vi "Stream Test.vi"() -> ()   [LabVIEW 2015]
uses:
  DAQ Engine VIs/PXI Globals.vi
panel:
  out "Graph":dbl[][](graph)
  out "Pause?":bool
  in  "Pause":bool
  in  "Gate":T1={"Active"=TRUE, "Delay (ms)"=20.0, "Width (ms)"=100.0, "Ramp (ms)"=5.0}
  out "Abort":bool
  in  "START":bool
  in  "RETURN":bool
  in  "STOP":bool
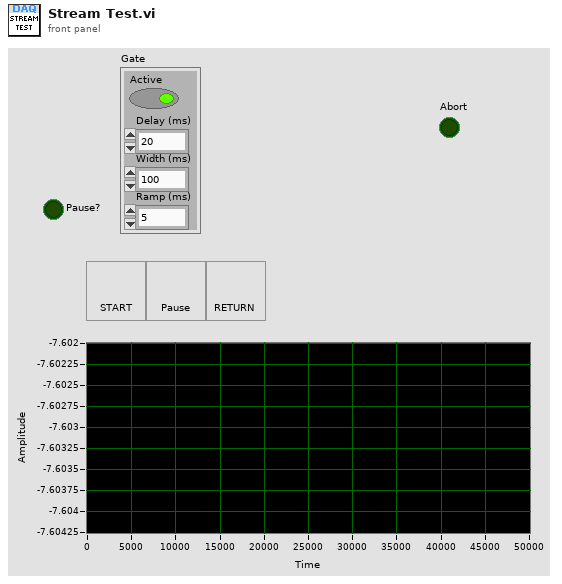
[diagram p1: front panel]
types:
  T1 = cluster{"Active":bool, "Delay (ms)":dbl, "Width (ms)":dbl, "Ramp (ms)":dbl}
  T2 = cluster{"Shift":bool, "Ctrl":bool, "Alt":bool, "Cmd":bool, "Opt":bool}
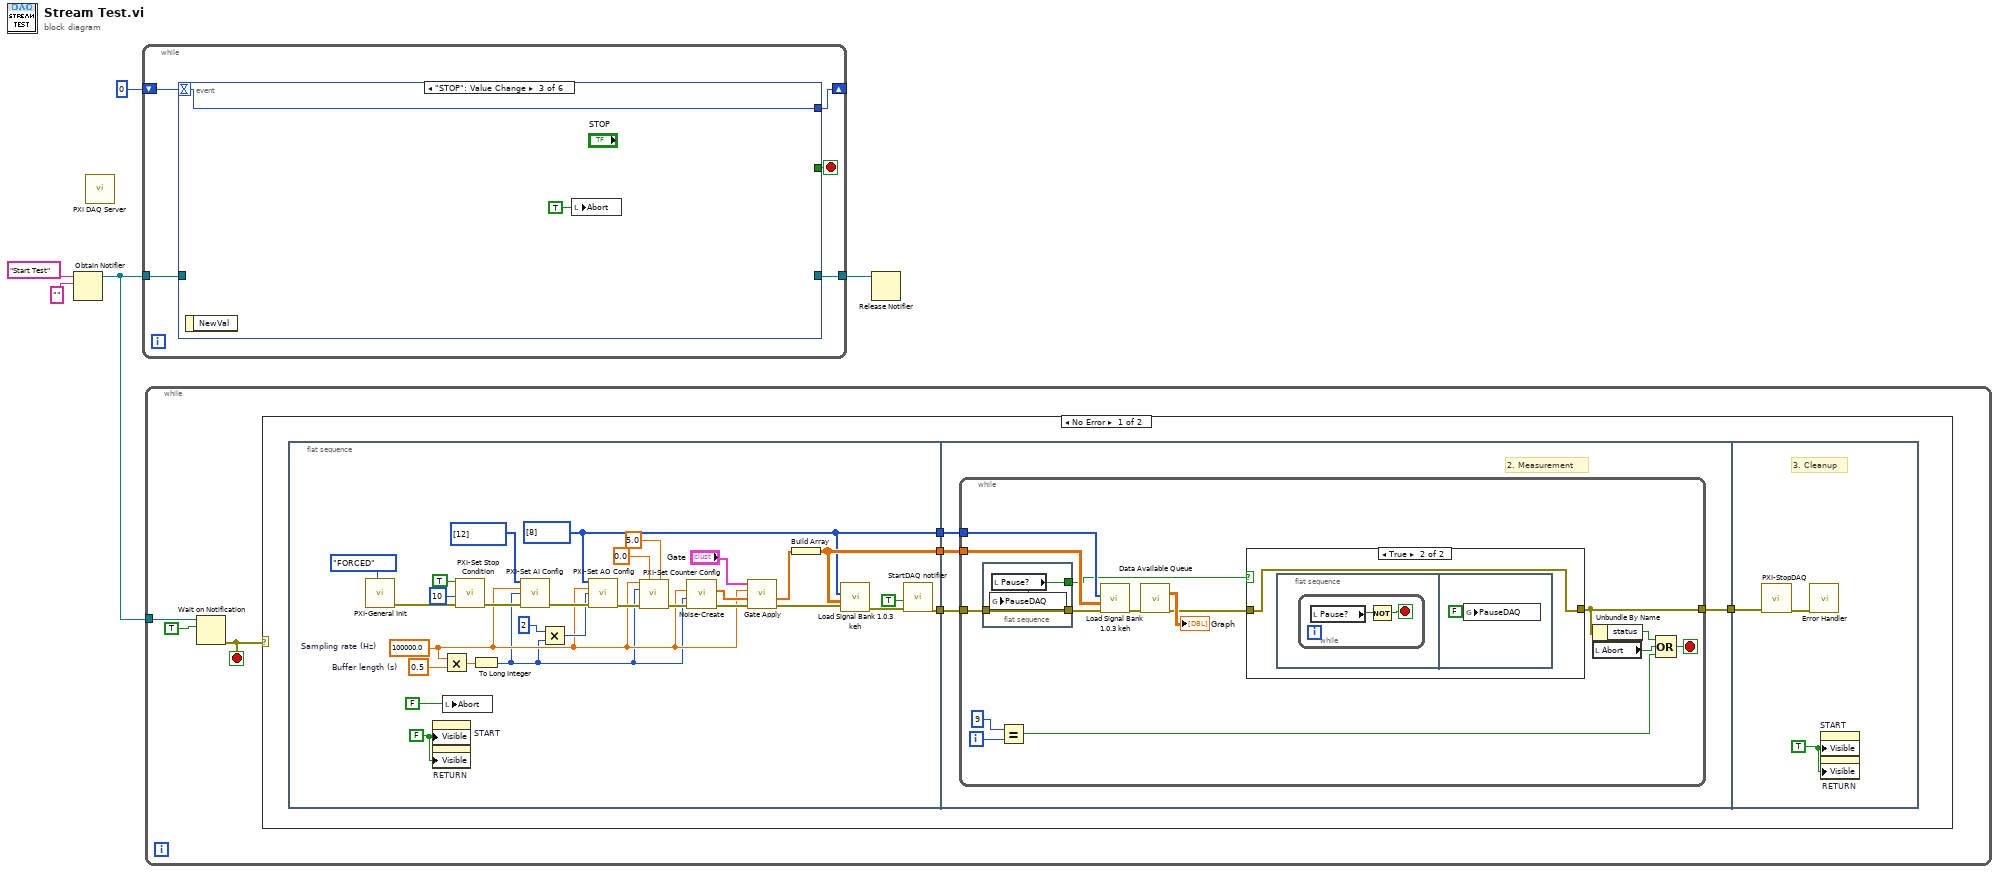
[diagram p0: block diagram]
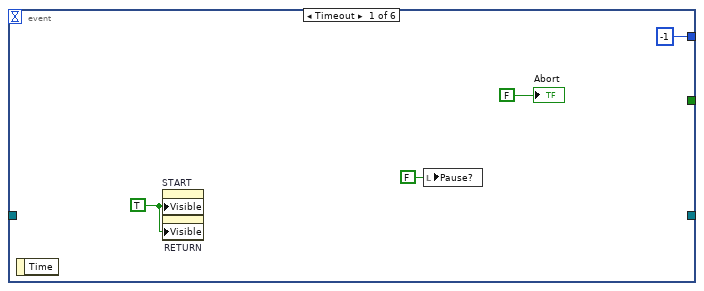
[diagram p4: hidden frame]
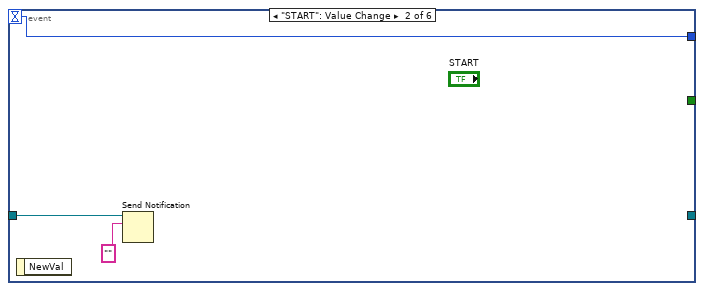
[diagram p5: hidden frame]
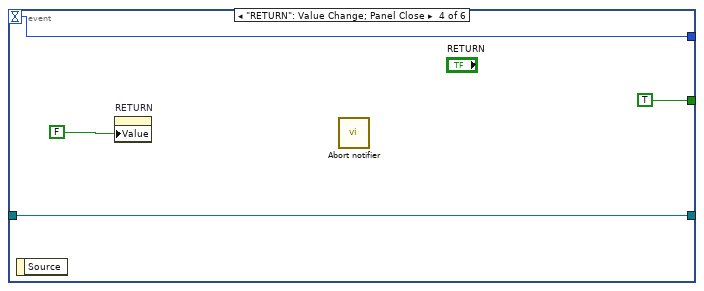
[diagram p6: hidden frame]
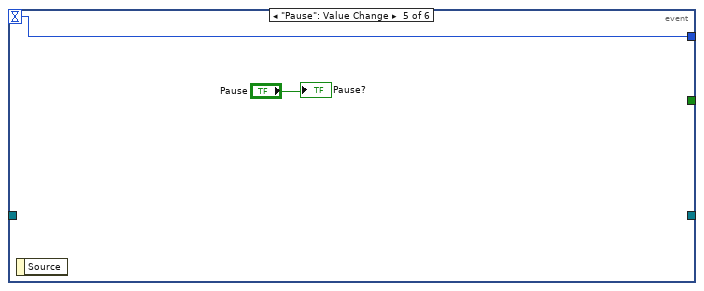
[diagram p7: hidden frame]
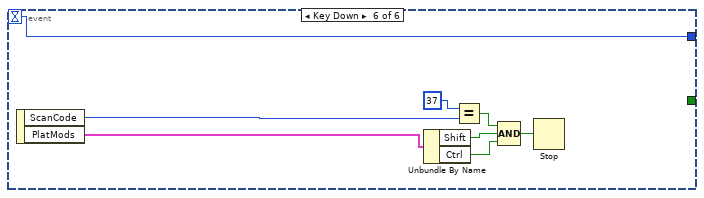
[diagram p8: hidden frame]
diagram:
  n1 = Obtain Notifier(name (unnamed)="Start Test", notification data type="") -> (notifier out=w5:refnum<notifier>)  [unwired: 2 in, 2 out]
  n2 = call "PXI DAQ Server.vi"() -> ()  [unwired: 7 in, 1 out]
  n3 = while {
    tunnel: w5 -> [w10]
    tunnel: [w8] -> w4
    shift-right: [w6] -> _
    shift-left: 0 -> [w7]
    stop <- w9 stop-if-true
    n4 = event shown="[2] \"STOP\": Value Change" {
      selector: _ -> [_ _ _ _ _ _]
      dyn-events: _ -> [_ _ _ _ _ _]
      timeout: w7 -> [_ w15 w18 w21 w25 w26]
      tunnel: w10 -> [_ w16 _ w22 _ _]
      tunnel: [_ _ _ TRUE _ _] -> w9
      tunnel: [_ _ _ w22 _ _] -> w8
      tunnel: [-1 w15 w18 w21 w25 w26] -> w6
      event Timeout {
        w12 = TRUE ("Visible")
        n5 = event-data() -> ()  [unwired: 1 in, 1 out]
        n6 = property on="START" class="Bool"("Visible"=w12) -> ()  [unwired: 2 in, 2 out]
        n7 = property on="RETURN" class="Bool (strict)"("Visible"=w12) -> ()  [unwired: 2 in, 2 out]
        n8 = local write "Pause?"(FALSE ("Pause?")) -> ()
        "Abort" <- FALSE ("Abort")
      }
      event "START": Value Change {
        n9 = event-data() -> ()  [unwired: 1 in, 1 out]
        n10 = Send Notification(notification="", notifier=w16) -> ()  [unwired: 1 in, 2 out]
      }
      event "STOP": Value Change {
        n11 = event-data() -> ()  [unwired: 1 in, 1 out]
        n12 = local write "Abort"(TRUE ("Global Abort")) -> ()
      }
      event "RETURN": Value Change; Panel Close {
        n13 = event-data() -> ()  [unwired: 1 in, 1 out]
        n14 = property on="RETURN" class="Bool (strict)"("Value"=FALSE) -> ()  [unwired: 2 in, 2 out]
        n15 = call "Abort notifier.vi"() -> ()  [unwired: 6 in, 2 out]
      }
      event "Pause": Value Change {
        n16 = event-data() -> ()  [unwired: 1 in, 1 out]
        "Pause?" <- "Pause"
      }
      event Key Down {
        n17 = event-data() -> ("ScanCode"=w28:i16, "PlatMods"=w27:T2)  [unwired: 1 in]
        n18 = Unbundle By Name(w27) -> ("Shift"=w31:bool, "Ctrl"=w30:bool)
        n19 = Equal?(x=i16 37 ("y"), y=w28) -> (x = y?=w32:bool)
        n20 = Compound Arithmetic op=AND(w32, w31, w30) -> (w29:bool)
        n21 = Stop(stop? (T)=w29) -> ()
      }
    }
  }
  n22 = while {
    tunnel: w5 -> [w35]
    stop <- w34 stop-if-true
    n23 = Wait on Notification(notifier=w35, ignore previous (F)=TRUE) -> (error out=w34:errorcluster)  [unwired: 2 in, 3 out]
    n24 = case shown="No Error" w34 {
      frame No Error {
        n25 = flat-sequence {
          tunnel: [w69] -> w40
          tunnel: [w49] -> w39
          tunnel: [w51] -> w38
          tunnel: w40 -> [w73]
          tunnel: w39 -> [w72]
          tunnel: w38 -> [w71]
          tunnel: [w70] -> w37
          tunnel: w37 -> [w96]
          frame #0 {
            w49 = i32[] [8] ("AI Channels")
            w58 = 0.5  # Buffer length (s)
            w44 = 100000.0  # Sampling rate (Hz)
            w68 = FALSE ("Visible")
            n26 = call "PXI-General Init.vi"("Double Buffer Mode"=enum32{"OFF", "ENABLED", "FORCED"}."FORCED") -> ("error out"=w59:errorcluster)  [unwired: 10 in]
            n27 = property on="START" class="Bool"("Visible"=w68) -> ()  [unwired: 2 in, 2 out]
            n28 = property on="RETURN" class="Bool (strict)"("Visible"=w68) -> ()  [unwired: 2 in, 2 out]
            n29 = Multiply(x=w44, y=w58) -> (x*y=w54:dbl)
            n30 = local write "Abort"(FALSE ("Global Abort")) -> ()
            n31 = call "PXI-Set Stop Condition.vi"("Stop on Max Presentations?"=TRUE, "Number of presentations"=10, "error in (no error)"=w59) -> ("error out"=w48:errorcluster)  [unwired: 12 in]
            n32 = To Long Integer(number=w54) -> (32bit integer=w43:i32)
            n33 = call "PXI-Set AI Config.vi"("AI Channels"=i32[] [12], "Sampling Rate (Hz)"=w44, "Buffer Size"=w43, "error in (no error)"=w48) -> ("error out"=w60:errorcluster)  [unwired: 11 in]
            n34 = Multiply(x=2, y=w43) -> (x*y=w56:i32)
            n35 = call "PXI-Set AO Config.vi"("AO Channels"=w49, "Sampling Rate (Hz)"=w44, "Buffer Size"=w56, "error in (no error)"=w60) -> ("error out"=w61:errorcluster)  [unwired: 11 in]
            n36 = call "PXI-Set Counter Config.vi"("AI Sampling Rate (Hz)"=w44, "Delay (ms)"=0.0, "pulse duration (ms)"=5.0, "Num AI Pts"=w43, "error in (no error)"=w61) -> ("error out"=w45:errorcluster)  [unwired: 10 in]
            n37 = call "Noise-Create.vi"("error in (no error)"=w45, "Npts"=w43, "Sampling Rate (Hz)"=w44) -> ("error out"=w62:errorcluster, "Waveform"=w63:dbl[])  [unwired: 6 in, 1 out]
            n38 = call "Gate Apply.vi"("error in (no error)"=w62, "Waveform in"=w63, "Sampling Rate (Hz)"=w44, "Gate Control"="Gate") -> ("error out"=w65:errorcluster, "Gated waveform"=w66:dbl[])  [unwired: 6 in]
            n39 = Build Array(w66) -> (w51:dbl[][])
            n40 = call "Load Signal Bank 1.0.3 keh.vi"("error in (no error)"=w65, "Input array"=w51, "Active AO Array"=w49) -> ("error out"=w53:errorcluster)  [unwired: 6 in, 2 out]
            n41 = call "StartDAQ notifier.vi"("error in (no error)"=w53, "wait for DAQ? (F)"=TRUE) -> ("error out"=w69:errorcluster)  [unwired: 5 in]
          }
          frame #1 {
            # "2. Measurement"
            n42 = while {
              tunnel: w73 -> [w79]
              tunnel: w72 -> [w86]
              tunnel: w71 -> [w85]
              tunnel: [w82] -> w70
              i -> [w76]
              stop <- w88 stop-if-true
              n43 = flat-sequence {
                tunnel: w79 -> [w90]
                tunnel: [w90] -> w78
                tunnel: [w89] -> w77
                frame #0 {
                  n44 = local read "Pause?"() -> (w89:bool)
                  n45 = global write "PXI Globals.vi" "PauseDAQ"(w89) -> ()
                }
              }
              n46 = Equal?(x=9, y=w76) -> (x = y?=w74:bool)
              n47 = call "Load Signal Bank 1.0.3 keh.vi"("error in (no error)"=w78, "Input array"=w85, "Active AO Array"=w86) -> ("error out"=w81:errorcluster)  [unwired: 6 in, 2 out]
              n48 = call "Data Available Queue.vi"("error in (no error)"=w81) -> ("Waveform Graph"=→"Graph":dbl[][], "error out"=w80:errorcluster)  [unwired: 10 in, 3 out]
              n49 = case shown="True" w77 {
                tunnel: w80 -> [w91 w92]
                tunnel: [w91 w92] -> w82
                frame False {
                }
                frame True {
                  n50 = flat-sequence {
                    frame #0 {
                      n51 = while {
                        stop <- w94 stop-if-true
                        n52 = local read "Pause?"() -> (w93:bool)
                        n53 = Not(x=w93) -> (.not. x?=w94:bool)
                      }
                    }
                    frame #1 {
                      n54 = global write "PXI Globals.vi" "PauseDAQ"(FALSE ("PauseDAQ")) -> ()
                    }
                  }
                }
              }
              n55 = Unbundle By Name(w82) -> ("status"=w84:bool)
              n56 = local read "Abort"() -> (w87:bool)
              n57 = Compound Arithmetic op=OR(w84, w87, w74) -> (w88:bool)
            }
          }
          frame #2 {
            w98 = TRUE ("Visible")
            # "3. Cleanup"
            n58 = call "PXI-StopDAQ.vi"("error in (no error)"=w96) -> ("error out"=w97:errorcluster)  [unwired: 6 in]
            n59 = call "Error Handler.vi"("error in (no error)"=w97) -> ()  [unwired: 13 in, 2 out]
            n60 = property on="START" class="Bool"("Visible"=w98) -> ()  [unwired: 2 in, 2 out]
            n61 = property on="RETURN" class="Bool (strict)"("Visible"=w98) -> ()  [unwired: 2 in, 2 out]
          }
        }
      }
      frame Error {
      }
    }
  }
  n62 = Release Notifier(notifier=w4) -> ()  [unwired: 2 in, 3 out]
